vi "util-io-csv-load.vi"(8 "error in":errorcluster, 11 "file path (dialog if empty)":path) -> (0 "error out":errorcluster, 3 "Array":T1[](array[typedef]) {"calibration"."Y" format="%#.3f"; "calibration"."X" format="%#.3f"; "ADDR" format="%04d"})   [LabVIEW 2024]
uses:
  controls/IONode.ctl
  controls/type.address.ctl
  controls/enum.io.type.ctl
  controls/enum.io.mode.ctl
  controls/typeXyPoint.ctl
  <vilib>/Utility/file.llb/Read Delimited Spreadsheet (string).vi
panel:
  out "array w/ subset deleted":string[][](array[string])
  out "headers":string[](array[string])
  # "Name\nType(AI,DI,DO,VL)\nMode(RIO,SIM)\nTags\nAddress (00-99)\nChannel (00-99)\nX1:Y1;X2:Y2"
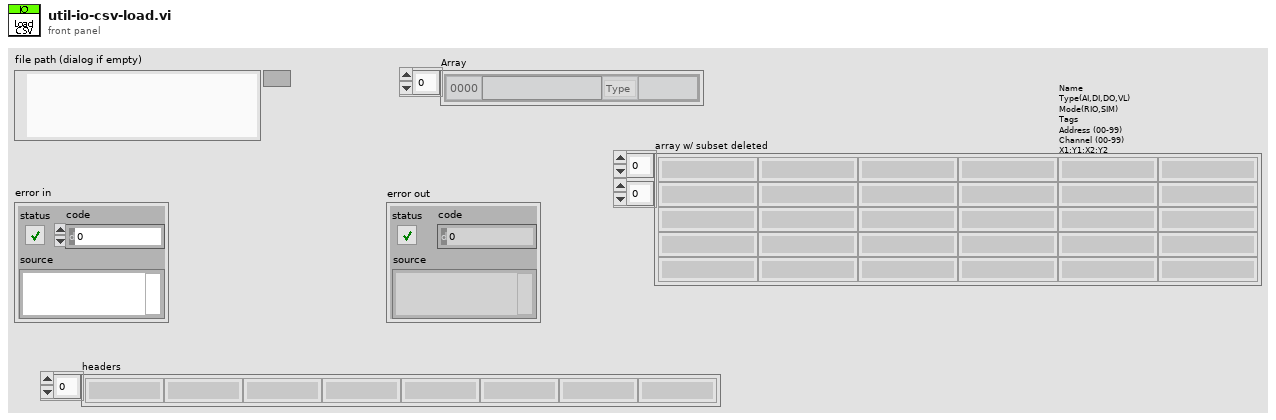
[diagram p1: front panel]
types:
  T1 = typedef "IONode.ctl" = cluster{"ADDR":T2, "Label":string, "Type":T3, "Mode":T4, "Value":string, "Tags":string, "calibration":T5[]}
  T2 = typedef "type.address.ctl" = u16
  T3 = typedef "enum.io.type.ctl" = enum16{"Type", "DI", "DO", "AI", "AO", "VL", "BUF"}
  T4 = typedef "enum.io.mode.ctl" = enum16{"Mode", "RIO", "SIM"}
  T5 = typedef "typeXyPoint.ctl" = cluster{"X":dbl, "Y":dbl}
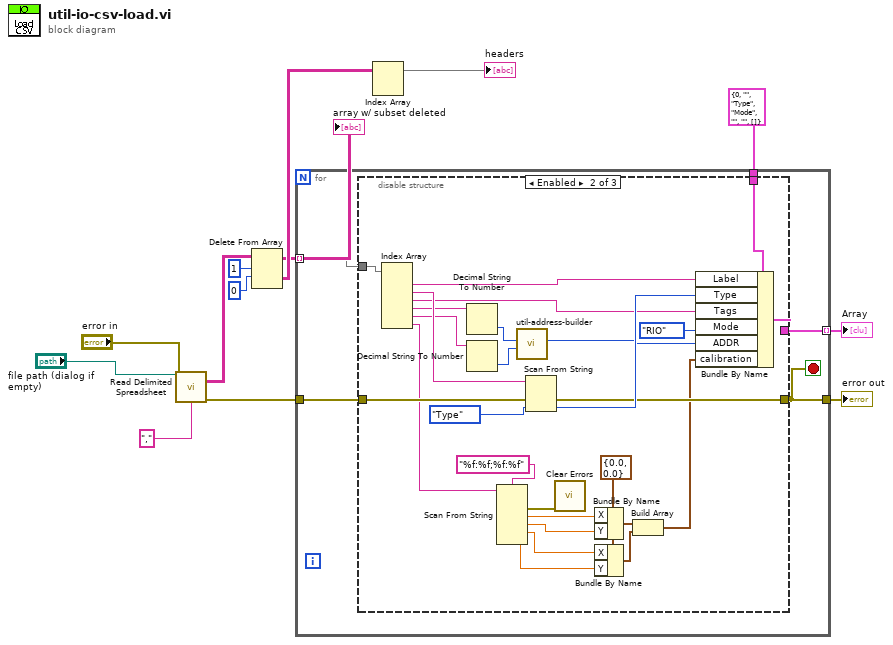
[diagram p0: block diagram]
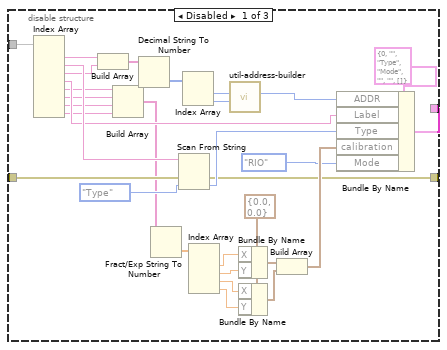
[diagram p2: hidden frame]
diagram:
  n1 = call-poly <vilib>:"Read Delimited Spreadsheet.vi"("file path (dialog if empty)"="file path (dialog if empty)", "error in (no error)"="error in", "delimiter (\\t)"="," ("delimiter (\\t)")) -> ("all rows"=w11:string[][], "error out"=w8:errorcluster)  [unwired: 7 in, 4 out]
  n2 = Delete From Array(array=w11, length=1, index (row)=0) -> (deleted portion=w6:string[][], array with subset deleted=w5:string[][])  [unwired: 1 in]
  "array w/ subset deleted" <- w5
  n3 = for {
    tunnel: [w18] -> w7 mode=indexing
    tunnel: w5 -> [w17] mode=indexing
    tunnel: [w15] -> w9
    tunnel: w8 -> [w16]
    tunnel: T1 {"ADDR"=0, "Label"="", "Type"=enum."Type", "Mode"=enum."Mode", "Value"="", "Tags"="", "calibration"=[]} ("IoConf in 3") -> [w14]
    stop <- w15 stop-if-true
    n4 = disable-structure shown="Enabled" {
      disable-tunnel: [w41 w74 _] -> w18
      disable-tunnel: w17 -> [w36 w70 _]
      disable-tunnel: w16 -> [w31 w68 _]
      disable-tunnel: [w30 w67 _] -> w15
      disable-tunnel: w14 -> [_ w65 _]
      frame Disabled {
        w40 = T5 {"X"=0.0, "Y"=0.0} ("calibration")
        n5 = Index Array(array=w36) -> (element #1=w35:string, element #2=w34:string, element #3=w33:string, element #4=w32:string, element #5=w29:string, element #6=w28:string, element #7=w27:string, element #8=w26:string)  [unwired: 8 in]
        n6 = Build Array(w35, w33) -> (w48:string[])
        n7 = Build Array(w29, w28, w27, w26) -> (w25:string[])
        n8 = Decimal String To Number(string=w48) -> (number=w47:i32[])  [unwired: 2 in, 1 out]
        n9 = Fract/Exp String To Number(string=w25) -> (number=w24:dbl[])  [unwired: 3 in, 1 out]
        n10 = Scan From String(input string=w34, error in=w31, default 1=enum.io.type."Type" ("type")) -> (error out=w30:errorcluster, output 1=w42:T3)  [unwired: 2 in, 2 out]
        n11 = Index Array(array=w47) -> (element #1=w46:i32, element #2=w45:i32)  [unwired: 2 in]
        n12 = Index Array(array=w24) -> (element #1=w23:dbl, element #2=w22:dbl, element #3=w21:dbl, element #4=w20:dbl)  [unwired: 4 in]
        n13 = call "util-address-builder.vi"("Channel"=w45, "Device"=w46) -> ("ADDR"=w44:T2)  [unwired: 9 in]
        n14 = Bundle By Name(cluster=w40, "X"=w23, "Y"=w22) -> (w39:T5)
        n15 = Bundle By Name(cluster=w40, "X"=w21, "Y"=w20) -> (w38:T5)
        n16 = Build Array(w39, w38) -> (w37:T5[])
        n17 = Bundle By Name(cluster=T1 {"ADDR"=0, "Label"="", "Type"=enum."Type", "Mode"=enum."Mode", "Value"="", "Tags"="", "calibration"=[]} ("IoConf in 3"), "ADDR"=w44, "Label"=w32, "Type"=w42, "calibration"=w37, "Mode"=enum.io.mode."RIO") -> (w41:T1)
      }
      frame Enabled {
        w73 = T5 {"X"=0.0, "Y"=0.0} ("calibration")
        n18 = Index Array(array=w70) -> (element #1=w64:string, element #2=w69:string, element #3=w63:string, element #4=w62:string, element #5=w61:string, element #6=w56:string)  [unwired: 6 in]
        n19 = Decimal String To Number(string=w62) -> (number=w60:i32)  [unwired: 2 in, 1 out]
        n20 = Decimal String To Number(string=w61) -> (number=w59:i32)  [unwired: 2 in, 1 out]
        n21 = Scan From String(format string="%f:%f;%f:%f", input string=w56) -> (error out=w50:errorcluster, output 1=w55:dbl, output 2=w54:dbl, output 3=w53:dbl, output 4=w52:dbl)  [unwired: 6 in, 2 out]
        n22 = call "util-address-builder.vi"("Channel"=w59, "Device"=w60) -> ("ADDR"=w58:T2)  [unwired: 9 in]
        n23 = Scan From String(input string=w69, error in=w68, default 1=enum.io.type."Type" ("type")) -> (error out=w67:errorcluster, output 1=w75:T3)  [unwired: 2 in, 2 out]
        n24 = call <vilib>:"Clear Errors.vi"("error in (no error)"=w50) -> ()  [unwired: 5 in, 2 out]
        n25 = Bundle By Name(cluster=w73, "X"=w55, "Y"=w54) -> (w72:T5)
        n26 = Bundle By Name(cluster=w73, "X"=w53, "Y"=w52) -> (w71:T5)
        n27 = Build Array(w72, w71) -> (w51:T5[])
        n28 = Bundle By Name(cluster=w65, "Label"=w64, "Type"=w75, "Tags"=w63, "Mode"=enum.io.mode."RIO", "ADDR"=w58, "calibration"=w51) -> (w74:T1)
      }
      frame Disabled {
      }
    }
  }
  "error out" <- w9
  "Array" <- w7
  n29 = Index Array(array=w6) -> (element=→"headers":string[])  [unwired: 2 in]
